vi "Reset Origin.vi"(6 "Variant in":variant, 7 "Shift Pressed?":bool, 8 "error in (no error)":errorcluster, 10 "QD Combo Box Ref":refnum<vi>, 11 "QD Launch VI Ref":refnum<vi>) -> (0 "error out":errorcluster, 4 "Variant out":variant)   [LabVIEW 2020, in "Control Operation.lvlib"]
doc: "Reset the origin of the front panel or block diagram to (0,0)."
uses:
  Control Operation.lvlib
  <vilib>/Utility/miscctls.llb/LVPointTypeDef.ctl
panel:
  in  "Undo Name":string="Reset to Origin"
  # "Do not change the connector pane of this VI.\n\nSee the block diagram for directions on how to use this template."
  # "Specify the name of the Undo transaction"
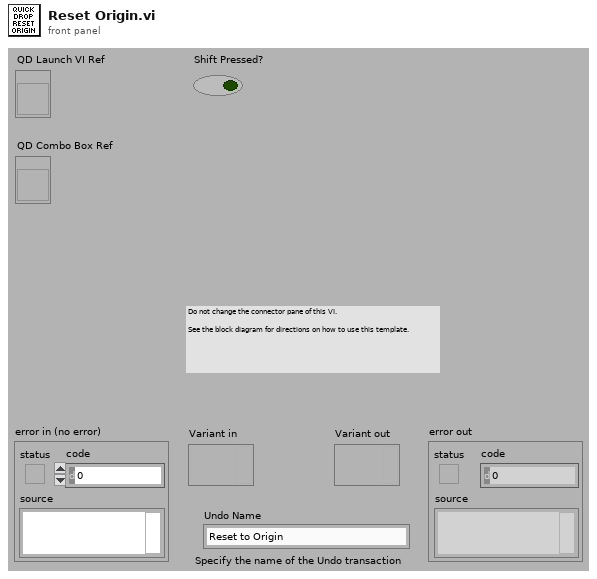
[diagram p1: front panel]
types:
  T1 = typedef "LVPointTypeDef.ctl" = cluster{"Horizontal":i16, "Vertical":i16}
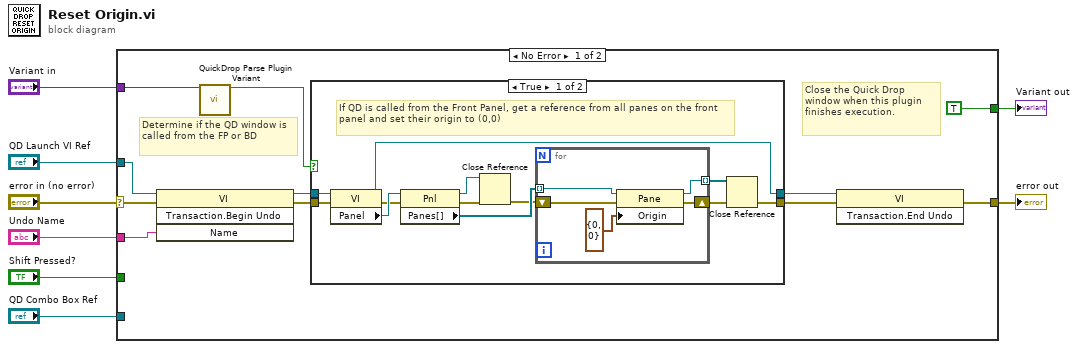
[diagram p0: block diagram]
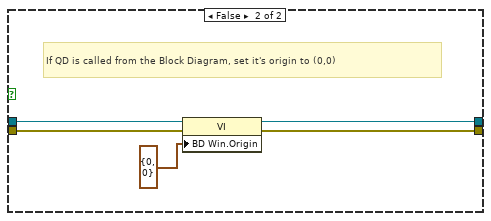
[diagram p2: hidden frame]
diagram:
  n1 = case shown="No Error" "error in (no error)" {
    selector: "error in (no error)" -> [w18 w42]
    tunnel: [w12 w42] -> w7
    tunnel: "QD Launch VI Ref" -> [w17 _]
    tunnel: "Shift Pressed?" -> [_ _]
    tunnel: "QD Combo Box Ref" -> [_ _]
    tunnel: "Variant in" -> [w19 _]
    tunnel: "Undo Name" -> [w16 _]
    tunnel: [TRUE _] -> w1
    frame No Error {
      # "Close the Quick Drop window when this plugin finishes execution."
      # "Determine if the QD window is called from the FP or BD"
      n2 = invoke class="VI" method="Transaction.Begin Undo"(reference=w17, error in=w18, "Name"=w16) -> (reference out=w11:refnum<vi>, error out=w13:errorcluster)  [unwired: 1 in, 2 out]
      n3 = call <vilib>:"QuickDrop Parse Plugin Variant.vi"("QDKS Variant in"=w19) -> ("QD Launch VI Panel?"=w14:bool)  [unwired: 12 in, 2 out]
      n4 = case shown="True" w14 {
        tunnel: w13 -> [w31 w39]
        tunnel: w11 -> [w30 w41]
        tunnel: [w21 w38] -> w10
        tunnel: [w20 w37] -> w9
        frame True {
          # "If QD is called from the Front Panel, get a reference from all panes on the front panel and set their origin to (0,0)"
          n5 = property class="VI"(reference=w30, error in=w31) -> (reference out=w20:refnum<vi>, error out=w27:errorcluster, "Panel"=w28:refnum<vi>)
          n6 = property class="Pnl"(reference=w28, error in=w27) -> (reference out=w23:refnum<vi>, error out=w24:errorcluster, "Panes[]"=w29:refnum<vi>[])
          n7 = Close Reference(reference=w23, error in (no error)=w24) -> (error out=w22:errorcluster)
          n8 = for {
            tunnel: w29 -> [w36] mode=indexing
            shift-right: [w33] -> w26
            shift-left: w22 -> [w34]
            tunnel: [w32] -> w25 mode=indexing
            n9 = property class="Pane"(reference=w36, error in=w34, "Origin"=T1 {"Horizontal"=0, "Vertical"=0}) -> (reference out=w32:refnum<vi>, error out=w33:errorcluster)
          }
          n10 = Close Reference(reference=w25, error in (no error)=w26) -> (error out=w21:errorcluster)
        }
        frame False {
          # "If QD is called from the Block Diagram, set it's origin to (0,0)"
          n11 = property class="VI"(reference=w41, error in=w39, "BD Win.Origin"=T1 {"Horizontal"=0, "Vertical"=0} ("Origin")) -> (reference out=w37:refnum<vi>, error out=w38:errorcluster)
        }
      }
      n12 = invoke class="VI" method="Transaction.End Undo"(reference=w9, error in=w10) -> (error out=w12:errorcluster)  [unwired: 1 in, 2 out]
    }
    frame Error {
    }
  }
  "error out" <- w7
  "Variant out" <- w1
